vi "Set IConfigure.vi"(8 "error in":errorcluster, 10 "IConfigure":refnum<class "IConfigure.lvclass">, 11 "IConfigurable in":refnum<class "IConfigurable.lvclass">) -> (0 "error out":errorcluster, 3 "IConfigurable out":refnum<class "IConfigurable.lvclass">)   [LabVIEW 2024, in "IConfigurable.lvclass"]
uses:
  IConfigurable.lvclass
  IConfigure/IConfigure.lvclass
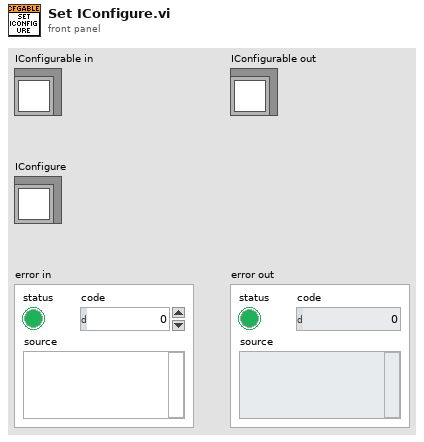
[diagram p1: front panel]
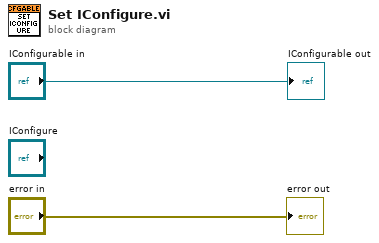
[diagram p0: block diagram]
diagram:
  "IConfigurable out" <- "IConfigurable in"
  "error out" <- "error in"
